vi "BuildMenu3.vi"(8 "Click Type":T1, 9 "Point":T2, 10 "XRef":refnum<vi>, 11 "State In":T10) -> (1 "Show Standard Items? (Popup click only)":bool=TRUE, 2 "Menu Specification":T4)   [LabVIEW 2018, in "ConPane Wrapper.xnode"]
uses:
  ConPane Wrapper.xnode
  State.ctl
  <vilib>/picture/picture.llb/imagedata.ctl
  <vilib>/XNodeSupport/XNodeTerm3Array.ctl
  <vilib>/XNodeSupport/XNodeTerm3.ctl
  <vilib>/XNodeSupport/XNodeString.ctl
  <vilib>/XNodeSupport/XNodeVariant.ctl
  <vilib>/XNodeSupport/XNodeRect32.ctl
  <vilib>/XNodeSupport/XNodeInt.ctl
  <vilib>/XNodeSupport/XNodeBool.ctl
  <vilib>/XNodeSupport/XNodeTermDirection.ctl
  Subvis/Term Types.ctl
  Subvis/Term Type.ctl
  <vilib>/XNodeSupport/XNodeMenuSpecs3.ctl
  <vilib>/XNodeSupport/XNodeMenuSpec3.ctl
  <vilib>/XNodeSupport/XNodeStandardHelpInfo.ctl
  <vilib>/XNodeSupport/XNodePath.ctl
  <vilib>/XNodeSupport/XNodePoint.ctl
  <vilib>/XNodeSupport/XNodeClickTypes.ctl
  <vilib>/XNodeSupport/NI_XNodeSupport.lvlib
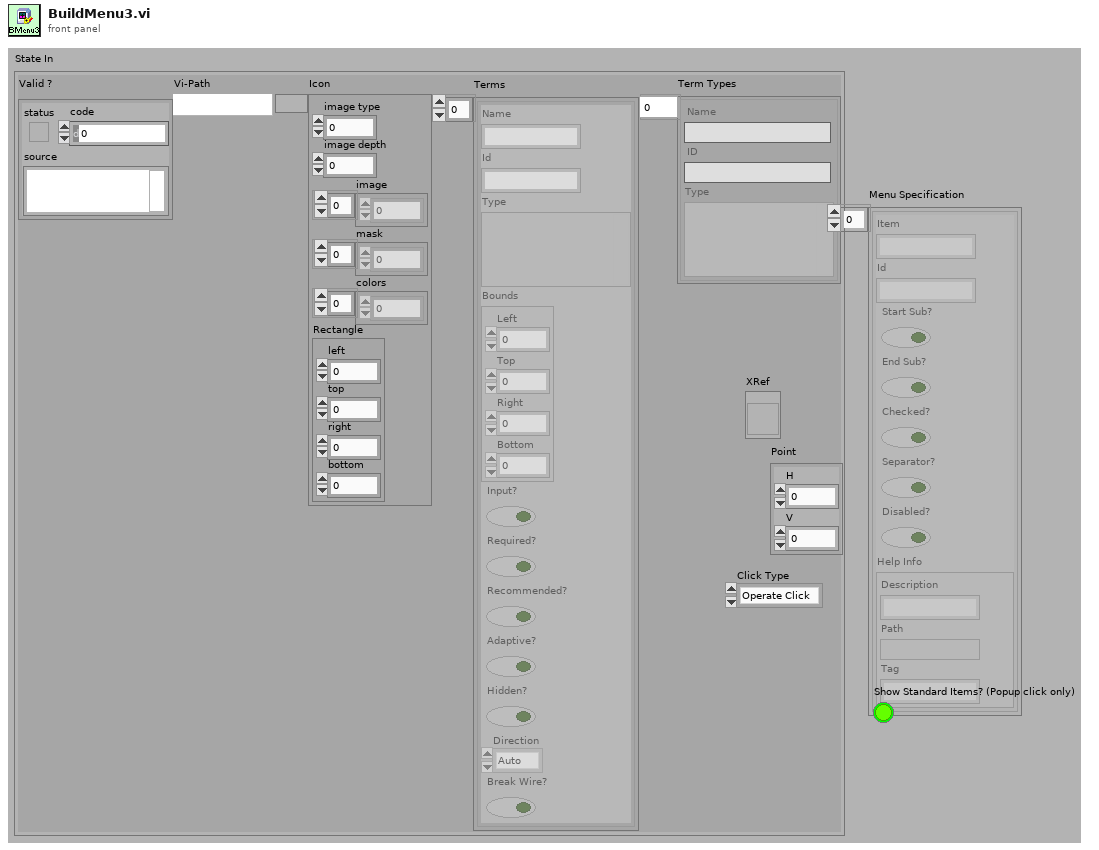
[diagram p1: front panel]
types:
  T1 = typedef "NI_XNodeSupport.lvlib/XNodeClickTypes.ctl" = enum32{"Operate Click", "Popup Click"}
  T2 = typedef "NI_XNodeSupport.lvlib/XNodePoint.ctl" = cluster{"H":T3, "V":T3}
  T3 = typedef "NI_XNodeSupport.lvlib/XNodeInt.ctl" = i32
  T4 = typedef "NI_XNodeSupport.lvlib/XNodeMenuSpecs3.ctl" = T5[]
  T5 = typedef "NI_XNodeSupport.lvlib/XNodeMenuSpec3.ctl" = cluster{"Item":T6, "Id":T6, "Start Sub?":T7, "End Sub?":T7, "Checked?":T7, "Separator?":T7, "Disabled?":T7, "Help Info":T8}
  T6 = typedef "NI_XNodeSupport.lvlib/XNodeString.ctl" = string
  T7 = typedef "NI_XNodeSupport.lvlib/XNodeBool.ctl" = bool
  T8 = typedef "NI_XNodeSupport.lvlib/XNodeStandardHelpInfo.ctl" = cluster{"Description":T6, "Path":T9, "Tag":T6}
  T9 = typedef "NI_XNodeSupport.lvlib/XNodePath.ctl" = path
  T10 = typedef "ConPane Wrapper.xnode/State.ctl" = cluster{"Valid ?":errorcluster, "Vi-Path":path, "Icon":T11, "Terms":T12, "Term Types":T17}
  T11 = typedef "imagedata.ctl" = cluster{"image type":i32, "image depth":i32, "image":u8[], "mask":u8[], "colors":u32[], "Rectangle":cluster{"left":i16, "top":i16, "right":i16, "bottom":i16}}
  T12 = typedef "NI_XNodeSupport.lvlib/XNodeTerm3Array.ctl" = T13[]
  T13 = typedef "NI_XNodeSupport.lvlib/XNodeTerm3.ctl" = cluster{"Name":T6, "Id":T6, "Type":T14, "Bounds":T15, "Input?":T7, "Required?":T7, "Recommended?":T7, "Adaptive?":T7, "Hidden?":T7, "Direction":T16, "Break Wire?":T7}
  T14 = typedef "NI_XNodeSupport.lvlib/XNodeVariant.ctl" = variant
  T15 = typedef "NI_XNodeSupport.lvlib/XNodeRect32.ctl" = cluster{"Left":T3, "Top":T3, "Right":T3, "Bottom":T3}
  T16 = typedef "NI_XNodeSupport.lvlib/XNodeTermDirection.ctl" = enum32{"Auto", "Up", "Down", "Left", "Right", "Center"}
  T17 = typedef "Term Types.ctl" = T18[]
  T18 = typedef "Term Type.ctl" = cluster{"Name":string, "ID":string, "Type":variant}
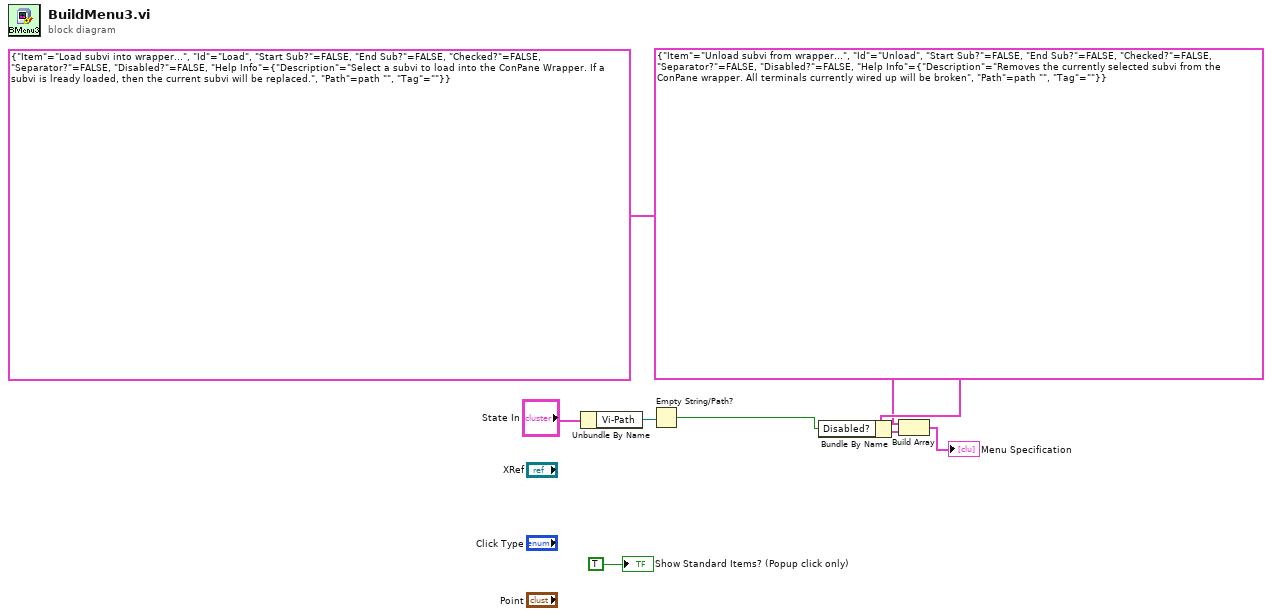
[diagram p0: block diagram]
diagram:
  n1 = Unbundle By Name("State In") -> ("Vi-Path"=w6:path)
  n2 = Empty String/Path?(string/path=w6) -> (empty?=w4:bool)
  n3 = Bundle By Name(cluster=T5 {"Item"="Unload subvi from wrapper...", "Id"="Unload", "Start Sub?"=FALSE, "End Sub?"=FALSE, "Checked?"=FALSE, "Separator?"=FALSE, "Disabled?"=FALSE, "Help Info"={"Description"="Removes the currently selected subvi from the ConPane wrapper. All terminals currently wired up will be broken", "Path"=path "", "Tag"=""}} ("Menu Item 3"), "Disabled?"=w4) -> (w3:T5)
  n4 = Build Array(T5 {"Item"="Load subvi into wrapper...", "Id"="Load", "Start Sub?"=FALSE, "End Sub?"=FALSE, "Checked?"=FALSE, "Separator?"=FALSE, "Disabled?"=FALSE, "Help Info"={"Description"="Select a subvi to load into the ConPane Wrapper. If a subvi is lready loaded, then the current subvi will be replaced.", "Path"=path "", "Tag"=""}} ("Menu Item 3"), w3) -> (→"Menu Specification":T5[])
  "Show Standard Items? (Popup click only)" <- TRUE ("Show Standard Items? (Popup click only)")
